vi "Relay Control.vi"(8 "error in (no error)":errorcluster, 9 "relay action (Close Relay)":T1=21 items=["Open Relay"=20, "Close Relay"=21], 10 "relay names":string, 11 "session in":T2) -> (0 "error out":errorcluster, 3 "session out":T2)   [LabVIEW 2020, in "SLSC Switch.lvlib"]
doc: "Controls individual relays of the switch module. When controlling individual relays, the protection offered by setting the usage of source channels and configurations channels is void."
uses:
  <vilib>/SLSC_Switch/SLSC Switch.lvlib
  nislscsl.dll
  <vilib>/userdefined/High Color/SLSC_Switch/nislscslSession.ctl
  <vilib>/SLSC_Switch/Relay Action.ctl
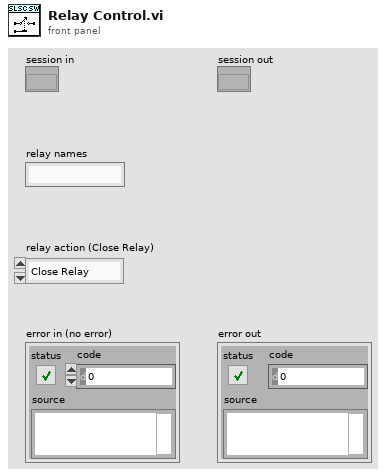
[diagram p1: front panel]
types:
  T1 = typedef "SLSC Switch.lvlib/Relay Action.ctl" = i32
  T2 = typedef "nislscslSession.ctl" = refnum<k20>
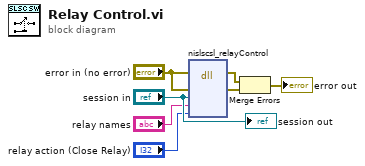
[diagram p0: block diagram]
diagram:
  n1 = dll-call lib="nislscsl.*" fn="nislscsl_relayControl"(error in="error in (no error)", "errorCluster"="error in (no error)", "sessionHandle"="session in", "connectionList"="relay names", "action"="relay action (Close Relay)") -> (error out=w7:errorcluster, "errorCluster"=w6:errorcluster)  [unwired: 6 in, 1 out]
  n2 = Merge Errors(w7, w6) -> (→"error out":errorcluster)
  "session out" <- "session in"
